vi "_Generate ControlDocMap.vi"(11 "Array":T1[](array[typedef])) -> (3 "Variant":variant)   [LabVIEW 2017, in "csmdoc.lvlib"]
uses:
  csmdoc.lvlib
  _Typedef/DocNote.ctl
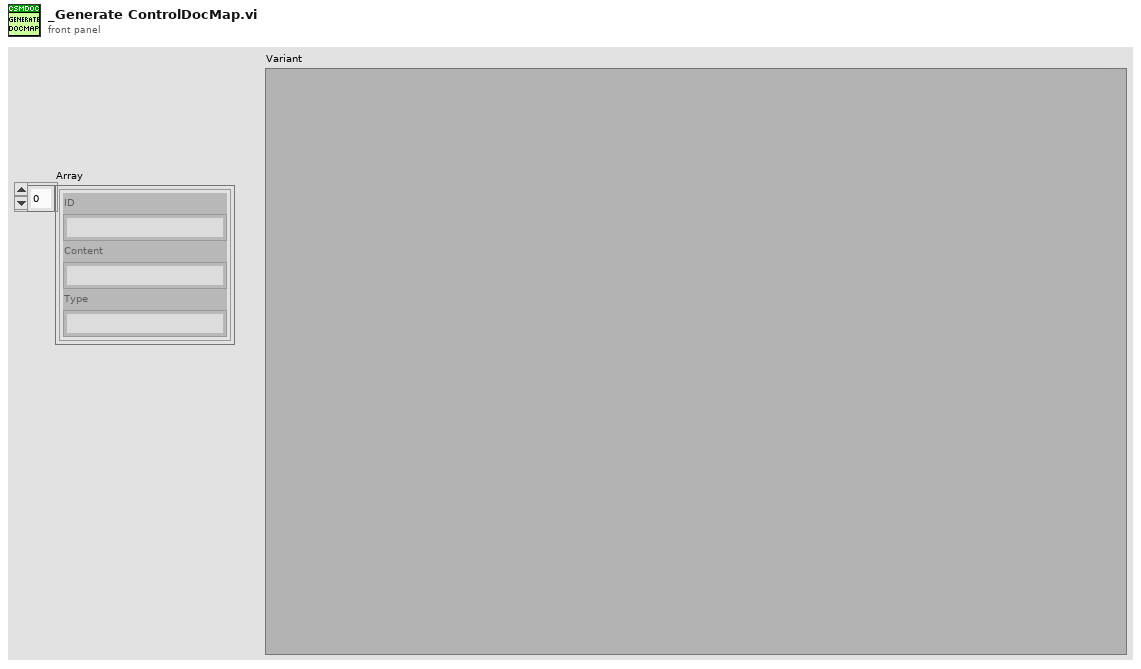
[diagram p1: front panel]
types:
  T1 = typedef "csmdoc.lvlib/DocNote.ctl" = cluster{"ID":string, "Content":string, "Type":string}
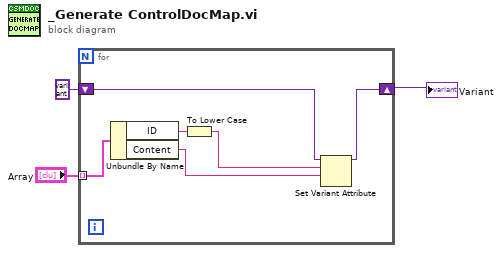
[diagram p0: block diagram]
diagram:
  n1 = for {
    tunnel: "Array" -> [w9] mode=indexing
    shift-right: [w7] -> w3
    shift-left: variant -> [w8]
    n2 = Unbundle By Name(w9) -> ("ID"=w6:string, "Content"=w4:string)
    n3 = To Lower Case(string=w6) -> (all lower case string=w5:string)
    n4 = Set Variant Attribute(Variant=w8, name=w5, value=w4) -> (Variant out=w7:variant)  [unwired: 1 in, 2 out]
  }
  "Variant" <- w3
